vi "shift_register.vi"() -> ()   [LabVIEW 2020]
panel:
  out "Cluster":T1
  out ".not. x?":bool[](array[boolean])
  out "Boolean":bool
  out "concatenated string":string
  out "Numeric":u16
  in  "stop":bool
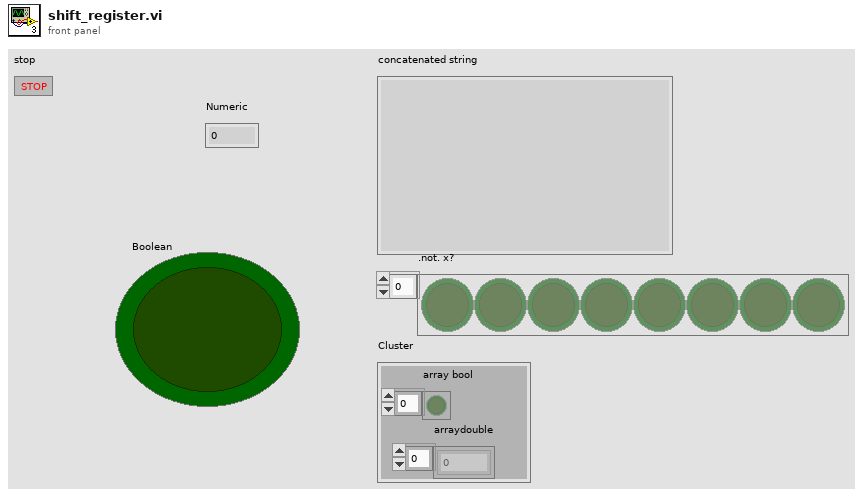
[diagram p1: front panel]
types:
  T1 = cluster{"array bool":bool[], "arraydouble":dbl[]}
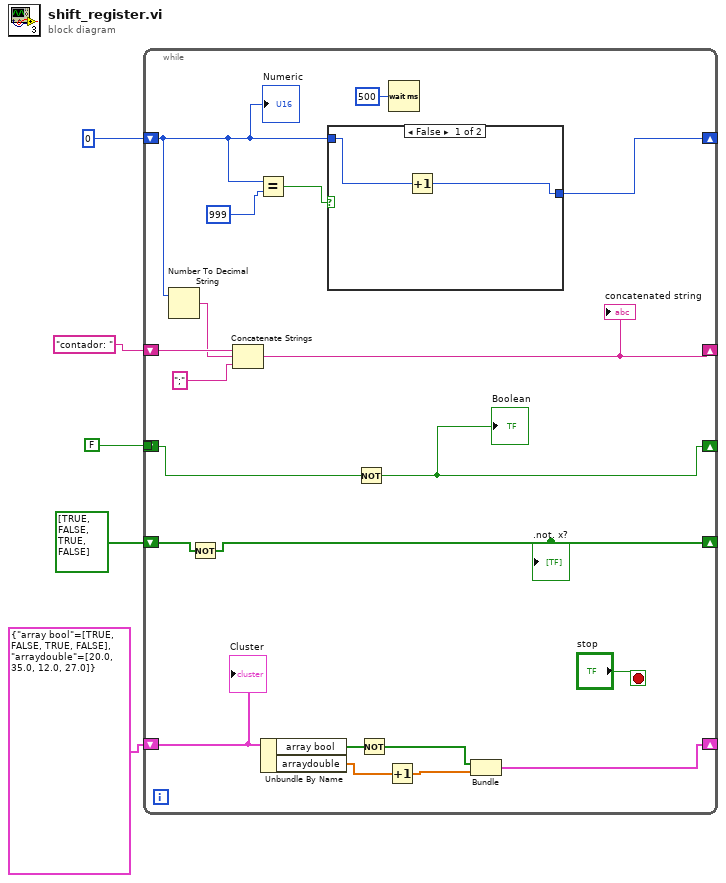
[diagram p0: block diagram]
diagram:
  n1 = while {
    shift-right: [w23] -> _
    shift-left: 0 -> [w19]
    shift-right: [w17] -> _
    shift-left: "contador: " -> [w20]
    tunnel: FALSE -> [_]
    shift-right: [w14] -> _
    shift-left: _ -> [w15]
    shift-right: [w12] -> _
    shift-left: bool[] [TRUE, FALSE, TRUE, FALSE] -> [w13]
    shift-right: [w6] -> _
    shift-left: T1 {"array bool"=[TRUE, FALSE, TRUE, FALSE], "arraydouble"=[20.0, 35.0, 12.0, 27.0]} -> [w11]
    stop <- "stop" stop-if-true
    n2 = Number To Decimal String(number=w19) -> (decimal integer string=w18:string)  [unwired: 1 in]
    n3 = Not(x=w13) -> (.not. x?=w12:bool[])
    ".not. x?" <- w12
    n4 = Concatenate Strings(w20, w18, ";") -> (w17:string)
    "concatenated string" <- w17
    n5 = Equal?(x=w19, y=999) -> (x = y?=w24:bool)
    n6 = Unbundle By Name(w11) -> ("array bool"=w10:bool[], "arraydouble"=w9:dbl[])
    n7 = case shown="False" w24 {
      tunnel: w19 -> [w27 w28]
      tunnel: [w26 w28] -> w23
      frame False {
        n8 = Increment(x=w27) -> (x+1=w26:i32)
      }
      frame True {
      }
    }
    n9 = Not(x=w15) -> (.not. x?=w14:bool)
    "Boolean" <- w14
    n10 = Not(x=w10) -> (.not. x?=w8:bool[])
    n11 = Increment(x=w9) -> (x+1=w7:dbl[])
    n12 = Wait (ms)(milliseconds to wait=u32 500) -> ()  [unwired: 1 out]
    n13 = Bundle(w8, w7) -> (w6:cluster{bool[], dbl[]})  [unwired: 1 in]
    "Numeric" <- w19
    "Cluster" <- w11
  }
